vi "MJSN_ClusterErrorToString.vi"(8 "Error In":errorcluster) -> (0 "Error Out":errorcluster, 1 "source string out":string, 2 "code string out":string, 3 "status string out":string)   [LabVIEW 2018]
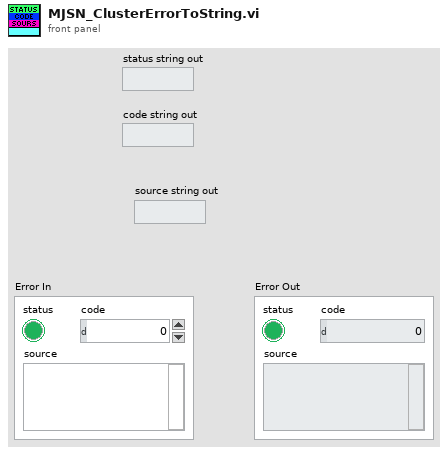
[diagram p1: front panel]
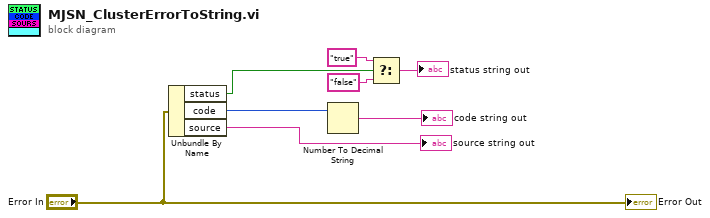
[diagram p0: block diagram]
diagram:
  n1 = Unbundle By Name("Error In") -> ("status"=w3:bool, "code"=w2:i32, "source"=→"source string out":string)
  n2 = Number To Decimal String(number=w2) -> (decimal integer string=→"code string out":string)  [unwired: 1 in]
  n3 = Select(t="true", s=w3, f="false") -> (s? t:f=→"status string out":string)
  "Error Out" <- "Error In"
